vi "SiosIfmSetRefMirrorVibration.vi"(1 "On / Off":i8(slide) scale=0.0..1.0, 2 "Channel":i32(knob) scale=1.0..4.0, 3 "Device Number":i32) -> (0 "Success":i32)   [LabVIEW 2009]
uses:
  siosifm.dll
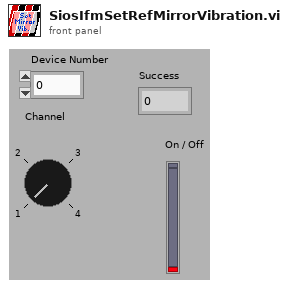
[diagram p1: front panel]
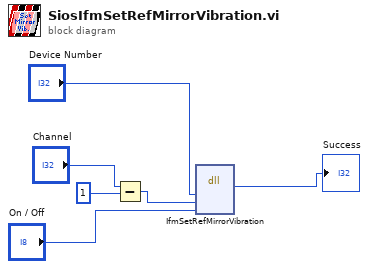
[diagram p0: block diagram]
diagram:
  n1 = Subtract(x="Channel", y=1) -> (x-y=w1:i32)
  n2 = dll-call lib="C:/WORK/Artem/RE-10/SIOS_IfmDLL/siosifm.dll" fn="IfmSetRefMirrorVibration"("devNumber"="Device Number", "channel"=w1, "on"="On / Off") -> ("success"=→"Success":i32)  [unwired: 6 in, 2 out]
